vi "Timer.vi"(10 "Stop Button":refnum<vi>, 11 "Gauge":refnum<vi>) -> ()   [LabVIEW 2011]
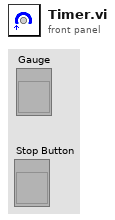
[diagram p1: front panel]
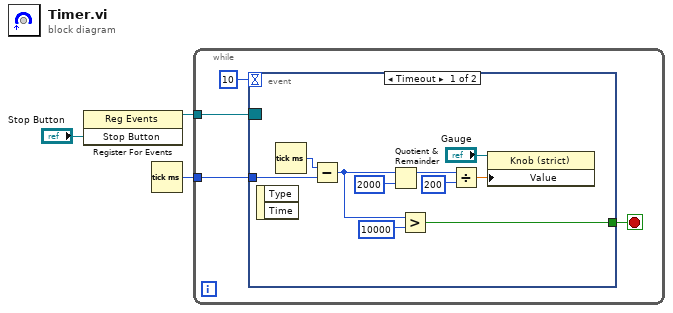
[diagram p0: block diagram]
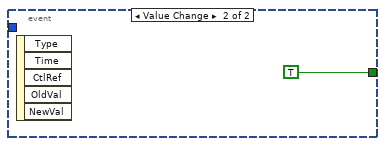
[diagram p2: hidden frame]
diagram:
  n1 = register-events("Stop Button") -> (reference out=w1:refnum<event-registration>)  [unwired: 2 in, 1 out]
  n2 = Tick Count (ms)() -> (millisecond timer value=w3:u32)
  n3 = while {
    tunnel: w3 -> [w7]
    tunnel: w1 -> [w4]
    stop <- w6 stop-if-true
    n4 = event shown="[0] Timeout" {
      selector: w4 -> [_ _]
      dyn-events: _ -> [_ _]
      timeout: 10 -> [_ _]
      tunnel: w7 -> [w16 _]
      tunnel: [w13 TRUE] -> w6
      event Timeout {
        n5 = event-data() -> ()  [unwired: 1 in, 2 out]
        n6 = Tick Count (ms)() -> (millisecond timer value=w17:u32)
        n7 = Subtract(x=w17, y=w16) -> (x-y=w12:u32)
        n8 = Quotient & Remainder(x=w12, y=u32 2000) -> (x-y*floor(x/y)=w10:u32)  [unwired: 1 out]
        n9 = Greater?(x=w12, y=u32 10000) -> (0:w13:bool)
        n10 = Divide(x=w10, y=u32 200) -> (x/y=w8:dbl)
        n11 = property class="Knob (strict)"(reference="Gauge", "Value"=w8) -> ()  [unwired: 1 in, 2 out]
      }
      event Value Change {
        n12 = event-data() -> ()  [unwired: 1 in, 5 out]
      }
    }
  }
